vi "Read Drive Joystick V.3.0.vi"(11 "JoystickDevRef":T1) -> ()   [LabVIEW 2017]
uses:
  <vilib>/Rock Robotics/WPI/Joystick/WPI_JoystickDevRef.ctl
  <vilib>/Rock Robotics/WPI/Joystick/WPI_JoystickDeviceEnum.ctl
  Robot Global Data V.3.0.vi
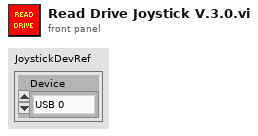
[diagram p1: front panel]
types:
  T1 = typedef "WPI_JoystickDevRef.ctl" = cluster{"Device":T2}
  T2 = typedef "WPI_JoystickDeviceEnum.ctl" = enum16{"USB 0", "USB 1", "USB 2", "USB 3", "USB 4", "USB 5"}
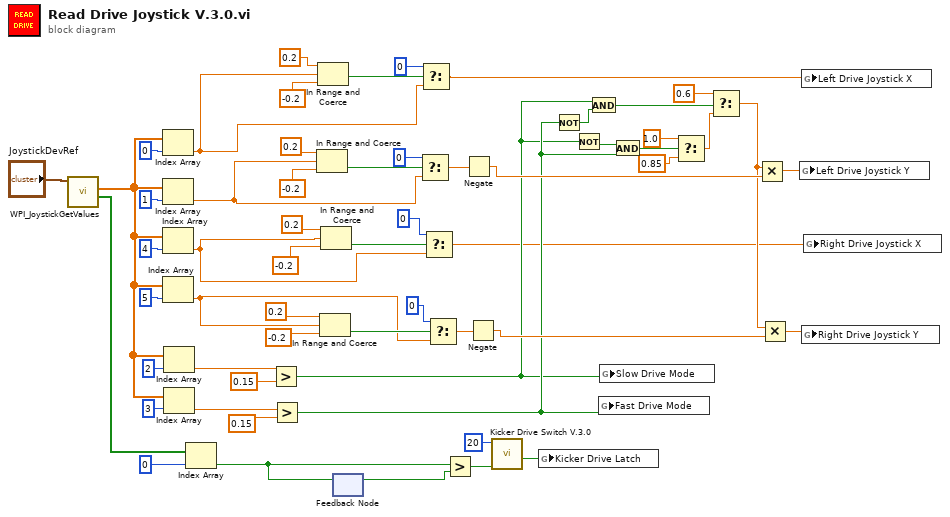
[diagram p0: block diagram]
diagram:
  n1 = call <vilib>:"WPI_JoystickGetValues.vi"("JoystickDevRef"="JoystickDevRef") -> ("Buttons"=w30:bool[], "Axes"=w22:dbl[])  [unwired: 6 in, 3 out]
  n2 = Index Array(array=w22, index=0) -> (element=w52:dbl)
  n3 = Index Array(array=w22, index=1) -> (element=w46:dbl)
  n4 = Index Array(array=w22, index=4) -> (element=w41:dbl)
  n5 = Index Array(array=w22, index=5) -> (element=w33:dbl)
  n6 = Index Array(array=w22, index=2) -> (element=w21:dbl)
  n7 = Index Array(array=w22, index=3) -> (element=w18:dbl)
  n8 = Index Array(array=w30, index=0) -> (element=w28:bool)
  n9 = Greater?(x=w21, y=0.15) -> (0:w8:bool)
  n10 = Greater?(x=w18, y=0.15) -> (0:w10:bool)
  n11 = In Range and Coerce(upper limit=0.2, x=w46, lower limit=-0.2) -> (In Range?=w48:bool)  [unwired: 1 out]
  n12 = In Range and Coerce(upper limit=0.2, x=w52, lower limit=-0.2) -> (In Range?=w53:bool)  [unwired: 1 out]
  n13 = In Range and Coerce(upper limit=0.2, x=w33, lower limit=-0.2) -> (In Range?=w37:bool)  [unwired: 1 out]
  n14 = In Range and Coerce(upper limit=0.2, x=w41, lower limit=-0.2) -> (In Range?=w42:bool)  [unwired: 1 out]
  n15 = feedback-in #1(w28) -> ()
  n16 = feedback #1() -> (w29:bool)  [unwired: 1 in]
  n17 = Select(t=0, s=w48, f=w46) -> (s? t:f=w47:dbl)
  n18 = Select(t=0, s=w53, f=w52) -> (s? t:f=w1:dbl)
  n19 = Select(t=0, s=w42, f=w41) -> (s? t:f=w2:dbl)
  n20 = Select(t=0, s=w37, f=w33) -> (s? t:f=w36:dbl)
  n21 = Greater?(x=w28, y=w29) -> (0:w27:bool)
  n22 = Negate(x=w47) -> (-x=w17:dbl)
  n23 = Negate(x=w36) -> (-x=w15:dbl)
  n24 = call "Kicker Drive Switch V.3.0.vi"("Input Button"=w27, "Time Until Reset"=20) -> ("On?"=w25:bool)  [unwired: 9 in]
  n25 = global write "Robot Global Data V.3.0.vi" "Kicker Drive Latch"(w25) -> ()
  n26 = Not(x=w10) -> (.not. x?=w13:bool)
  n27 = Not(x=w8) -> (.not. x?=w9:bool)
  n28 = And(x=w8, y=w13) -> (x .and. y?=w12:bool)
  n29 = global write "Robot Global Data V.3.0.vi" "Fast Drive Mode"(w10) -> ()
  n30 = global write "Robot Global Data V.3.0.vi" "Slow Drive Mode"(w8) -> ()
  n31 = And(x=w9, y=w10) -> (x .and. y?=w7:bool)
  n32 = Select(t=1.0, s=w7, f=0.85) -> (s? t:f=w4:dbl)
  n33 = Select(t=0.6, s=w12, f=w4) -> (s? t:f=w3:dbl)
  n34 = Multiply(x=w3, y=w17) -> (x*y=w14:dbl)
  n35 = Multiply(x=w3, y=w15) -> (x*y=w16:dbl)
  n36 = global write "Robot Global Data V.3.0.vi" "Left Drive Joystick Y"(w14) -> ()
  n37 = global write "Robot Global Data V.3.0.vi" "Left Drive Joystick X"(w1) -> ()
  n38 = global write "Robot Global Data V.3.0.vi" "Right Drive Joystick Y"(w16) -> ()
  n39 = global write "Robot Global Data V.3.0.vi" "Right Drive Joystick X"(w2) -> ()
